vi "Excute.vi"(8 "error in (no error)":errorcluster, 11 "Cmd3 in":refnum<class "Cmd3.lvclass">) -> (0 "error out":errorcluster, 3 "Cmd3 out":refnum<class "Cmd3.lvclass">)   [LabVIEW 2014, in "Cmd3.lvclass"]
uses:
  Cmd3.lvclass
  Worker1/Worker1(receiver).lvclass
  Worker2/Worker2(receiver).lvclass
  Worker3/Worker3(receiver).lvclass
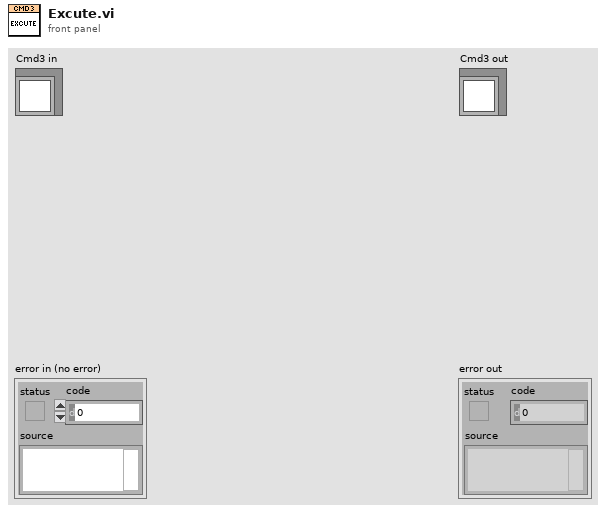
[diagram p1: front panel]
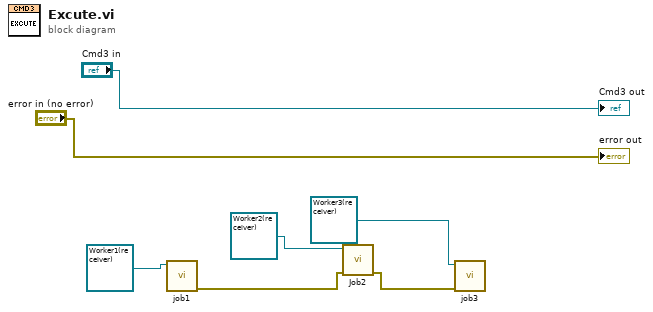
[diagram p0: block diagram]
diagram:
  n1 = call "job1.vi"("Worker1(receiver) in"=refnum<class "Worker1(receiver).lvclass"> refnum ("Worker1(receiver).lvclass")) -> ("error out"=w4:errorcluster)  [unwired: 9 in, 1 out]
  n2 = call "Job2.vi"("error in (no error)"=w4, "Worker2(receiver) in"=refnum<class "Worker2(receiver).lvclass"> refnum ("Worker2(receiver).lvclass")) -> ("error out"=w5:errorcluster)  [unwired: 8 in, 1 out]
  n3 = call "job3.vi"("error in (no error)"=w5, "Worker3(receiver) in"=refnum<class "Worker3(receiver).lvclass"> refnum ("Worker3(receiver).lvclass")) -> ()  [unwired: 8 in, 2 out]
  "error out" <- "error in (no error)"
  "Cmd3 out" <- "Cmd3 in"
